vi "displayControlElement.vi"(10 "viewThisComponent":refnum<class "ViewThisComponent.lvclass">) -> ()   [LabVIEW 2016, in "EXAViewElements.lvlib"]
doc: "Displays a control element."
uses:
  EXAViewElements.lvlib
  ViewThisComponent/ViewThisComponent.lvclass
  home/andres/ct_cmpuserevents/ComponentTemplateCore/ComponentModel/ComponentModel/View/View.lvclass
  ComponentTemplateCore/Hyperlink/Hyperlink.ctl
  Typedefs/StateValue.ctl
  Typedefs/SubDataSignal.ctl
  displayControlElement2.vi
  Typedefs/EXATypedefs.lvlib
  ComponentTemplateCore/ComponentModel/ComponentModel/View/View.lvclass
panel:
  in  "Show me":T1
  in  "sendAValueIsTrue":bool caption="Start"
  in  "aValue":dbl[unit] format="%.2f"
  in  "DoThisIsTrue":bool caption="Start"
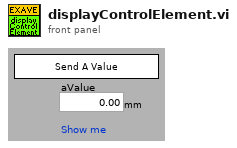
[diagram p1: front panel]
types:
  T1 = typedef "Hyperlink.ctl" = bool
  T2 = typedef "TypedefsDataEvents.lvlib/PubDataEvents.ctl" = cluster{"AppliedSettingsMatchStart":refnum<user-event>, "SettingVersions":refnum<user-event>, "SummaryState":refnum<user-event>, "RejectedCommand":refnum<user-event>, "DetailedState":refnum<user-event>, "ErrorCode":refnum<user-event>, "Heartbeat":refnum<user-event>, "LoopTime_ms":refnum<user-event>, "LoopTimeOutOfRange":refnum<user-event>, "Timestamp":refnum<user-event>}
  T3 = typedef "EXATypedefs.lvlib/StateValue.ctl" = enum16{"", " DisabledState", "EnabledState", "FaultState", "OfflineState", "StandbyState"}
  T4 = typedef "EXATypedefs.lvlib/SubDataSignal.ctl" = enum16{"Disable", "Enable", "Exit", "GoToStandby", "HeartbeatIn", "Start"}
  T5 = enum16{"", " DisabledState", "EnabledState", "FaultState", "OfflineState", "StandbyState"}
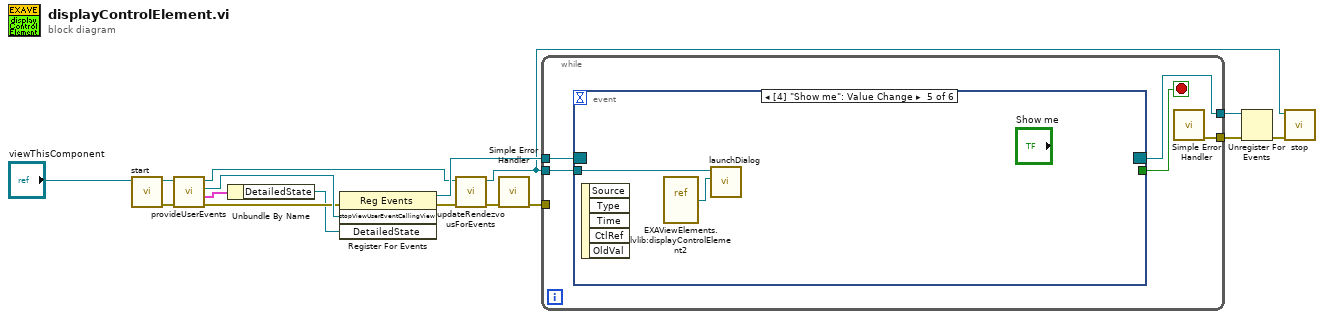
[diagram p0: block diagram]
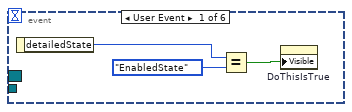
[diagram p2: hidden frame]
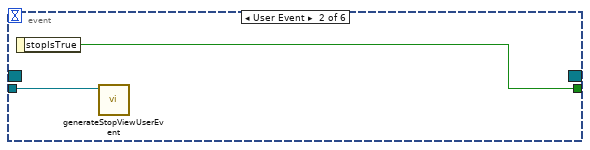
[diagram p3: hidden frame]
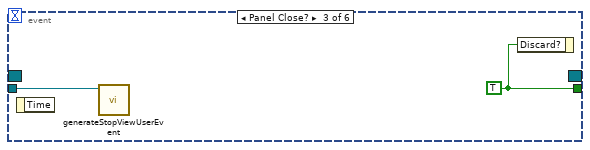
[diagram p4: hidden frame]
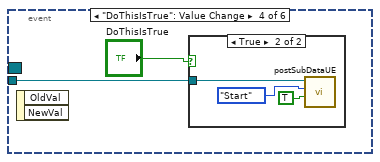
[diagram p5: hidden frame]
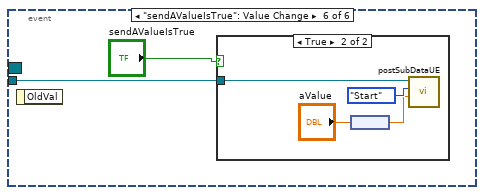
[diagram p7: hidden frame]
diagram:
  n1 = call-dynamic "start.vi"("View in"="viewThisComponent") -> ("error out"=w7:errorcluster, "View out"=w12:refnum<class "ViewThisComponent.lvclass">)  [unwired: 9 in]
  n2 = call "provideUserEvents.vi"("error in (no error)"=w7, "ViewThisComponent in"=w12) -> ("error out"=w13:errorcluster, "pubDataEvents"=w14:T2, "stopViewUserEventCallingView"=w15:refnum<user-event>, "ViewThisComponent out"=w2:refnum<class "ViewThisComponent.lvclass">)  [unwired: 6 in]
  n3 = Unbundle By Name(w14) -> ("DetailedState"=w10:refnum<user-event>)
  n4 = register-events(error in=w13, w15, w10) -> (reference out=w11:refnum<event-registration>, error out=w4:errorcluster)  [unwired: 1 in]
  n5 = call "updateRendezvousForEvents.vi"("error in (no error)"=w4, "View in"=w2) -> ("error out"=w3:errorcluster, "View out"=w1:refnum<class "ViewThisComponent.lvclass">)  [unwired: 8 in]
  n6 = call <vilib>:"Simple Error Handler.vi"("error in (no error)"=w3) -> ("error out"=w5:errorcluster)  [unwired: 4 in, 4 out]
  n7 = while {
    tunnel: w11 -> [w21]
    tunnel: w1 -> [w20]
    tunnel: [w19] -> w6
    tunnel: [w17] -> w9
    tunnel: w5 -> [_]
    stop <- w18 stop-if-true
    n8 = event shown="[4] \"Show me\": Value Change" {
      selector: w21 -> [_ _ _ _ _ _]
      dyn-events: [_ _ _ _ _ _] -> w17
      timeout: _ -> [_ _ _ _ _ _]
      tunnel: w20 -> [_ w25 w28 w29 w34 w36]
      tunnel: [_ w26 w27 _ _ _] -> w18
      event User Event {
        n9 = event-data() -> ("detailedState"=w22:T5)  [unwired: 1 in]
        n10 = Equal?(x=w22, y=StateValue."EnabledState" ("StateValue")) -> (x = y?=w23:bool)
        n11 = property on="DoThisIsTrue" class="Bool"("Visible"=w23) -> ()  [unwired: 2 in, 2 out]
      }
      event User Event {
        n12 = event-data() -> ("stopIsTrue"=w26:bool)  [unwired: 1 in]
        n13 = call "generateStopViewUserEvent.vi"("View in"=w25) -> ()  [unwired: 9 in, 2 out]
      }
      event Panel Close? {
        w27 = TRUE ("Discard?")
        n14 = event-data() -> ()  [unwired: 1 in, 1 out]
        n15 = call "generateStopViewUserEvent.vi"("View in"=w28) -> ()  [unwired: 9 in, 2 out]
        n16 = event-data("Discard?"=w27) -> ()  [unwired: 1 in, 1 out]
      }
      event "DoThisIsTrue": Value Change {
        n17 = event-data() -> ()  [unwired: 1 in, 2 out]
        n18 = case shown="True" "DoThisIsTrue" {
          tunnel: w29 -> [_ w31]
          frame False {
          }
          frame True {
            n19 = call "postSubDataUE.vi"("value"=TRUE ("Start"), "subDataSV"=SubDataSignal."Start" ("SubDataSV"), "ViewThisComponent in"=w31) -> ()  [unwired: 7 in, 2 out]
          }
        }
      }
      event Value Change {
        n20 = event-data() -> ()  [unwired: 1 in, 5 out]
        n21 = vi-ref "EXAViewElements.lvlib:displayControlElement2.vi"() -> (w35:refnum<vi>)
        n22 = call "launchDialog.vi"("dialogVIRefnum"=w35, "View in"=w34) -> ()  [unwired: 8 in, 2 out]
      }
      event "sendAValueIsTrue": Value Change {
        n23 = event-data() -> ()  [unwired: 1 in, 1 out]
        n24 = case shown="True" "sendAValueIsTrue" {
          tunnel: w36 -> [_ w38]
          frame False {
          }
          frame True {
            n25 = node("aValue") -> (w39:dbl)
            n26 = call "postSubDataUE.vi"("value"=w39, "subDataSV"=SubDataSignal."Start" ("SubDataSV"), "ViewThisComponent in"=w38) -> ()  [unwired: 7 in, 2 out]
          }
        }
      }
    }
    n27 = call <vilib>:"Simple Error Handler.vi"() -> ("error out"=w19:errorcluster)  [unwired: 5 in, 4 out]
  }
  n28 = Unregister For Events(event registration refnum=w9, error in=w6) -> (error out=w8:errorcluster)
  n29 = call-dynamic "stop.vi"("error in (no error)"=w8, "View in"=w1) -> ()  [unwired: 8 in, 2 out]
